vi "Excel Report - Generate from Template.vi"() -> ()   [LabVIEW 2023]
doc: "This example shows how to generate a report from a template. The template contains a preformatted table and a preformatted graph which are updated with Append Table to Report.vi and Excel Update Graph.vi."
uses:
  <vilib>/Utility/NIReport.llb/Report Type.ctl
  <vilib>/Utility/NIReport.llb/Append Report Text (str wrap).vi
  <vilib>/Utility/NIReport.llb/Append Text Table to Report (wrap).vi
  <vilib>/Utility/NIReport.llb/NI_report.lvclass
  <vilib>/Utility/NIReport.llb/Excel/NI_Excel.lvclass
  <vilib>/Utility/NIReport.llb/NI_ReportGenerationCore.lvlib
panel:
  in  "Express VI?":bool
  in  "Test operator":string="Operator's name"
  in  "Pressure":string="100"
  in  "Humidity":string="70"
  in  "Temperature":string="20"
  in  "Data":string[][](table)=[["100", "41.7", "38.5"], ["125", "41.7", "35.2"], ["160", "41.5", "37.5"], ["200", "42.3", "42.5"], ["250", "46.9", "46.8"], ["315", "51.9", "52.6"], ["400", "52.3", "46.7"], ["500  ", "46.5", "41.6"], ["630", "42.3", "35.9"], ["800", "41.1", "32.6"]]
  # "Overview: This example shows how to generate a report from a template using either the Excel Report Generation VIs or the MS Office Report Express VI.\nRequirements: Report Generation Toolkit, Microsoft Excel\nInstructions:\nRun the VI."
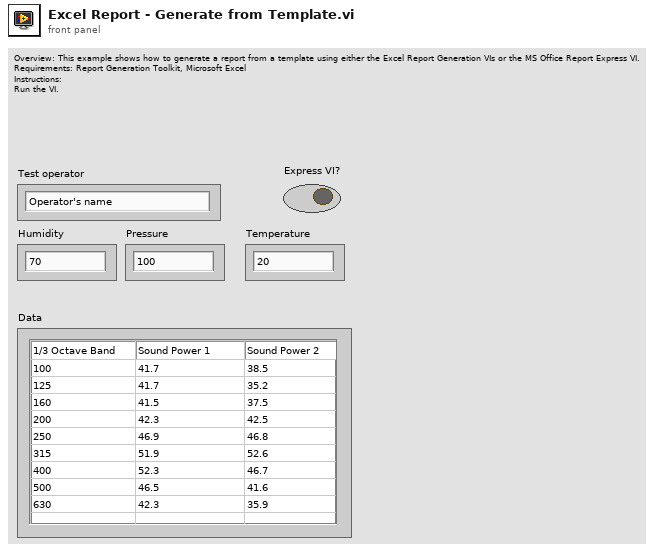
[diagram p1: front panel]
types:
  T1 = typedef "NI_ReportGenerationCore.lvlib/Report Type.ctl" = enum16{"HTML", "Word", "Excel"}
  T2 = cluster{"position (Excel)":cluster{"row":i32, "column":i32}, "name (Excel)":string, "bookmark (Word)":string}
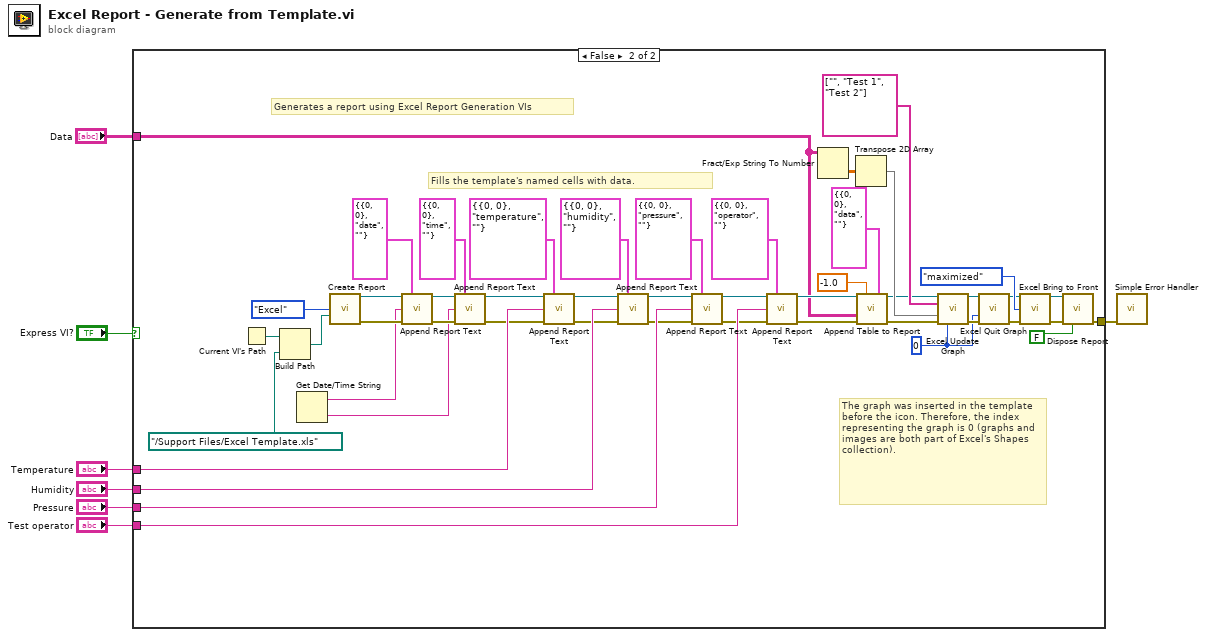
[diagram p0: block diagram]
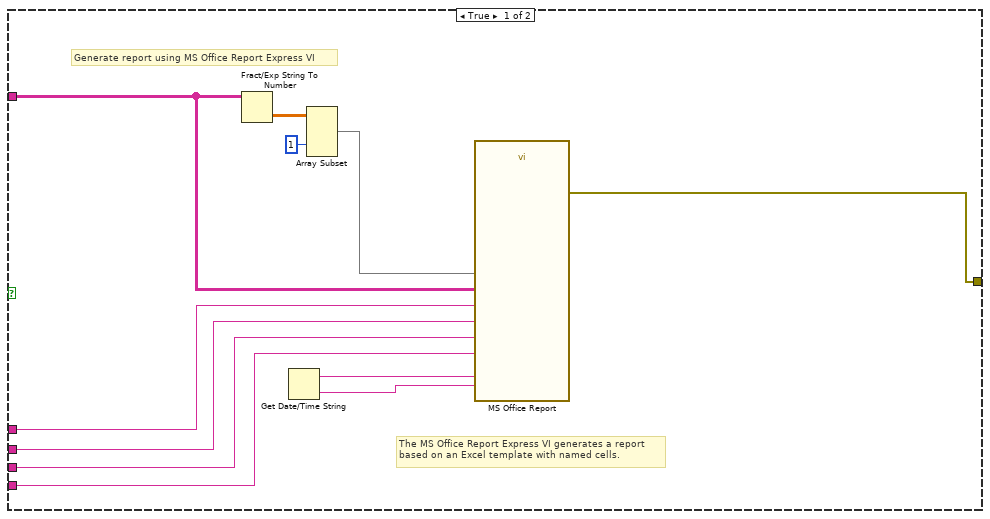
[diagram p2: hidden frame]
diagram:
  n1 = case shown="False" "Express VI?" {
    tunnel: "Temperature" -> [w13 w66]
    tunnel: "Humidity" -> [w12 w65]
    tunnel: "Pressure" -> [w11 w64]
    tunnel: "Test operator" -> [w10 w63]
    tunnel: [w14 w62] -> w3
    tunnel: "Data" -> [w15 w21]
    frame True {
      # "Generate report using MS Office Report Express VI"
      # "The MS Office Report Express VI generates a report\nbased on an Excel template with named cells."
      n2 = Fract/Exp String To Number(string=w15) -> (number=w18:dbl[][])  [unwired: 3 in, 1 out]
      n3 = Get Date/Time String() -> (date string=w9:string, time string=w8:string)  [unwired: 3 in]
      n4 = Array Subset(array=w18, index (col)=1 ("index")) -> (w16:dbl[][])  [unwired: 3 in]
      n5 = call "MS Office Report"("chart"=w16, "data"=w15, "date"=w9, "humidity"=w12, "operator"=w10, "pressure"=w11, "temperature"=w13, "time"=w8) -> ("error out"=w14:errorcluster)  [unwired: 19 in]
    }
    frame False {
      w39 = i16 0 ("graph index")
      # "Fills the template's named cells with data."
      # "The graph was inserted in the template before the icon. Therefore, the index representing the graph is 0 (graphs and images are both part of Excel's Shapes collection)."
      # "Generates a report using Excel Report Generation VIs"
      n6 = Current VI's Path() -> (path=w22:path)
      n7 = Build Path(base path=w22, name or relative path=path "../Support Files/Excel Template.xls") -> (appended path=w47:path)
      n8 = Get Date/Time String() -> (date string=w23:string, time string=w24:string)  [unwired: 3 in]
      n9 = call <vilib>:"Create Report.vi"("report type"=Report_Type."Excel" ("Report Type"), "template (empty)"=w47) -> ("report out"=w54:refnum<class "NI_report.lvclass">, "error out"=w60:errorcluster)  [unwired: 12 in]
      n10 = call-poly <vilib>:"Append Report Text.vi"("report in"=w54, "MS Office parameters"=T2 {"position (Excel)"={"row"=0, "column"=0}, "name (Excel)"="date", "bookmark (Word)"=""}, "text"=w23, "error in (no error)"=w60) -> ("report out"=w53:refnum<class "NI_report.lvclass">, "error out"=w59:errorcluster)  [unwired: 8 in, 2 out]
      n11 = call-poly <vilib>:"Append Report Text.vi"("report in"=w53, "MS Office parameters"=T2 {"position (Excel)"={"row"=0, "column"=0}, "name (Excel)"="time", "bookmark (Word)"=""}, "text"=w24, "error in (no error)"=w59) -> ("report out"=w52:refnum<class "NI_report.lvclass">, "error out"=w58:errorcluster)  [unwired: 8 in, 2 out]
      n12 = call-poly <vilib>:"Append Report Text.vi"("report in"=w52, "MS Office parameters"=T2 {"position (Excel)"={"row"=0, "column"=0}, "name (Excel)"="temperature", "bookmark (Word)"=""}, "text"=w66, "error in (no error)"=w58) -> ("report out"=w51:refnum<class "NI_report.lvclass">, "error out"=w57:errorcluster)  [unwired: 8 in, 2 out]
      n13 = call-poly <vilib>:"Append Report Text.vi"("report in"=w51, "MS Office parameters"=T2 {"position (Excel)"={"row"=0, "column"=0}, "name (Excel)"="humidity", "bookmark (Word)"=""}, "text"=w65, "error in (no error)"=w57) -> ("report out"=w50:refnum<class "NI_report.lvclass">, "error out"=w56:errorcluster)  [unwired: 8 in, 2 out]
      n14 = call-poly <vilib>:"Append Report Text.vi"("report in"=w50, "MS Office parameters"=T2 {"position (Excel)"={"row"=0, "column"=0}, "name (Excel)"="pressure", "bookmark (Word)"=""}, "text"=w64, "error in (no error)"=w56) -> ("report out"=w49:refnum<class "NI_report.lvclass">, "error out"=w55:errorcluster)  [unwired: 8 in, 2 out]
      n15 = call-poly <vilib>:"Append Report Text.vi"("report in"=w49, "MS Office parameters"=T2 {"position (Excel)"={"row"=0, "column"=0}, "name (Excel)"="operator", "bookmark (Word)"=""}, "text"=w63, "error in (no error)"=w55) -> ("report out"=w36:refnum<class "NI_report.lvclass">, "error out"=w35:errorcluster)  [unwired: 8 in, 2 out]
      n16 = Fract/Exp String To Number(string=w21) -> (number=w61:dbl[][])  [unwired: 3 in, 1 out]
      n17 = Transpose 2D Array(2D array=w61) -> (transposed array=w37:dbl[][])
      n18 = call-poly <vilib>:"Append Table to Report.vi"("report in"=w36, "column width (1)"=-1.0, "MS Office parameters"=T2 {"position (Excel)"={"row"=0, "column"=0}, "name (Excel)"="data", "bookmark (Word)"=""}, "text data"=w21, "error in (no error)"=w35) -> ("report out"=w34:refnum<class "NI_report.lvclass">, "error out"=w33:errorcluster)  [unwired: 7 in, 2 out]
      n19 = call <vilib>:"Excel Update Graph.vi"("report in"=w34, "row header"=string[] ["", "Test 1", "Test 2"], "graph data"=w37, "error in (no error)"=w33, "graph index (-1)"=w39) -> ("report out"=w41:refnum<class "NI_report.lvclass">, "error out"=w40:errorcluster)  [unwired: 9 in]
      n20 = call <vilib>:"Excel Quit Graph.vi"("report in"=w41, "graph index (-1)"=w39, "error in (no error)"=w40) -> ("report out"=w42:refnum<class "NI_report.lvclass">, "error out"=w43:errorcluster)  [unwired: 11 in]
      n21 = call <vilib>:"Excel Bring to Front.vi"("report in"=w42, "window state (maximized)"=enum16{"maximized", "minimized", "normal"}."maximized", "error in (no error)"=w43) -> ("report out"=w46:refnum<class "NI_report.lvclass">, "error out"=w45:errorcluster)  [unwired: 11 in]
      n22 = call-dynamic "Dispose Report.vi"("report in"=w46, "error in (no error)"=w45, "close report? (T)"=FALSE ("Close Report? (T)")) -> ("error out"=w62:errorcluster)  [unwired: 12 in]
    }
  }
  n23 = call <vilib>:"Simple Error Handler.vi"("error in (no error)"=w3) -> ()  [unwired: 4 in, 5 out]
